vi "Siglent SPD3000 Series Output.vi"() -> ()   [LabVIEW 2015]
doc: "This example shows how to configure the instrument's output voltage, output current and return the actual voltage level and actual current level."
uses:
  <instrlib>/Siglent SPD3000 Series/Siglent SPD3000 Series.lvlib
panel:
  out "Actual Current Level (A)":dbl
  out "Actual Voltage Level (V)":dbl
  out "Actual Current Level (A)":dbl
  out "Actual Voltage Level (V)":dbl
  in  "Current Setting (0 A)":dbl min=0.0 max=3.2 format="%.3f"
  in  "Voltage Setting (0 V)":dbl min=0.0 max=32.0 format="%.3f"
  in  "Current Setting (0 A)":dbl min=0.0 max=3.2 format="%.3f"
  in  "Voltage Setting (0 V)":dbl min=0.0 max=32.0 format="%.3f"
  in  "Stop Output":bool
  in  "VISA resource name":refnum<visa-resource-name>
  # "(c) 2016 SIGLENT TECHNOLOGIES CO., LTD.   ALL RIGHTS RESERVED."
  # "Channel"
  # "Channe2"
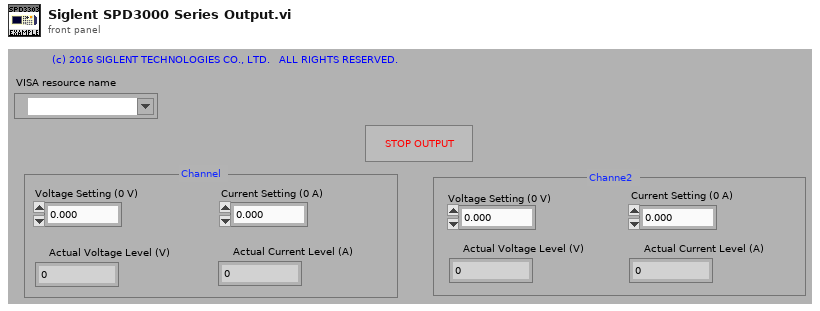
[diagram p1: front panel]
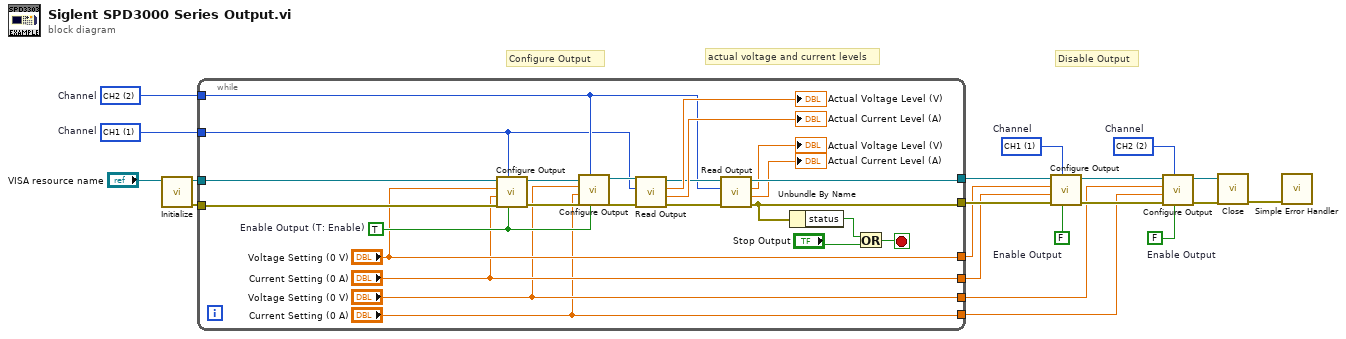
[diagram p0: block diagram]
diagram:
  w1 = u16 2 items=["CH1"=1, "CH2"=2]  # Channel
  w2 = u16 1 items=["CH1"=1, "CH2"=2]  # Channel
  w7 = FALSE  # Enable Output
  w13 = FALSE  # Enable Output
  w15 = u16 2 items=["CH1"=1, "CH2"=2]  # Channel
  w14 = u16 1 items=["CH1"=1, "CH2"=2]  # Channel
  # "actual voltage and current levels"
  # "Disable Output"
  # "Configure Output"
  n1 = call <instrlib>:"Initialize.vi"("VISA resource name"="VISA resource name") -> ("error out"=w19:errorcluster, "VISA resource name out"=w20:refnum<visa-resource-name>)  [unwired: 9 in]
  n2 = while {
    tunnel: w20 -> [w30]
    tunnel: w19 -> [w27]
    tunnel: [w37] -> w17
    tunnel: [w36] -> w16
    tunnel: w15 -> [w31]
    tunnel: w14 -> [w26]
    tunnel: ["Voltage Setting (0 V)"] -> w6
    tunnel: ["Current Setting (0 A)"] -> w5
    tunnel: ["Voltage Setting (0 V)"] -> w4
    tunnel: ["Current Setting (0 A)"] -> w3
    stop <- w44 stop-if-true
    w25 = TRUE  # Enable Output (T: Enable)
    n3 = call <instrlib>:"Configure Output.vi"("Enable Output (T: Enable)"=w25, "Channel (1:CH1)"=w26, "error in (no error)"=w27, "Current (0 A)"="Current Setting (0 A)", "Voltage (0 V)"="Voltage Setting (0 V)", "VISA resource name"=w30) -> ("error out"=w28:errorcluster, "VISA resource name out"=w29:refnum<visa-resource-name>)  [unwired: 4 in]
    n4 = call <instrlib>:"Configure Output.vi"("Enable Output (T: Enable)"=w25, "Channel (1:CH1)"=w31, "error in (no error)"=w28, "Current (0 A)"="Current Setting (0 A)", "Voltage (0 V)"="Voltage Setting (0 V)", "VISA resource name"=w29) -> ("error out"=w32:errorcluster, "VISA resource name out"=w33:refnum<visa-resource-name>)  [unwired: 4 in]
    n5 = call <instrlib>:"Read Output.vi"("error in (no error)"=w32, "Channel (1: CH1)"=w26, "VISA resource name"=w33) -> ("error out"=w39:errorcluster, "Actual Current Level (A)"=→"Actual Current Level (A)":dbl, "Actual Voltage Level (V)"=→"Actual Voltage Level (V)":dbl, "VISA resource name out"=w38:refnum<visa-resource-name>)  [unwired: 5 in]
    n6 = call <instrlib>:"Read Output.vi"("error in (no error)"=w39, "Channel (1: CH1)"=w31, "VISA resource name"=w38) -> ("error out"=w36:errorcluster, "Actual Current Level (A)"=→"Actual Current Level (A)":dbl, "Actual Voltage Level (V)"=→"Actual Voltage Level (V)":dbl, "VISA resource name out"=w37:refnum<visa-resource-name>)  [unwired: 5 in]
    n7 = Unbundle By Name(w36) -> ("status"=w40:bool)
    n8 = Or(x=w40, y="Stop Output") -> (x .or. y?=w44:bool)
  }
  n9 = call <instrlib>:"Configure Output.vi"("Enable Output (T: Enable)"=w13, "Channel (1:CH1)"=w2, "error in (no error)"=w16, "Current (0 A)"=w5, "Voltage (0 V)"=w6, "VISA resource name"=w17) -> ("error out"=w10:errorcluster, "VISA resource name out"=w11:refnum<visa-resource-name>)  [unwired: 4 in]
  n10 = call <instrlib>:"Configure Output.vi"("Enable Output (T: Enable)"=w7, "Channel (1:CH1)"=w1, "error in (no error)"=w10, "Current (0 A)"=w3, "Voltage (0 V)"=w4, "VISA resource name"=w11) -> ("error out"=w8:errorcluster, "VISA resource name out"=w9:refnum<visa-resource-name>)  [unwired: 4 in]
  n11 = call <instrlib>:"Close.vi"("error in (no error)"=w8, "VISA resource name"=w9) -> ("error out"=w12:errorcluster)  [unwired: 9 in]
  n12 = call <vilib>:"Simple Error Handler.vi"("error in (no error)"=w12) -> ()  [unwired: 4 in, 5 out]
